vi "MALT132_0001.vi"() -> ()   [LabVIEW 2018]
uses:
  <instrlib>/AltonTech MALT/AltonTech MALT200817.lvlib
panel:
  in  "K1":bool
  in  "stop":bool
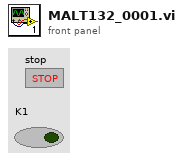
[diagram p1: front panel]
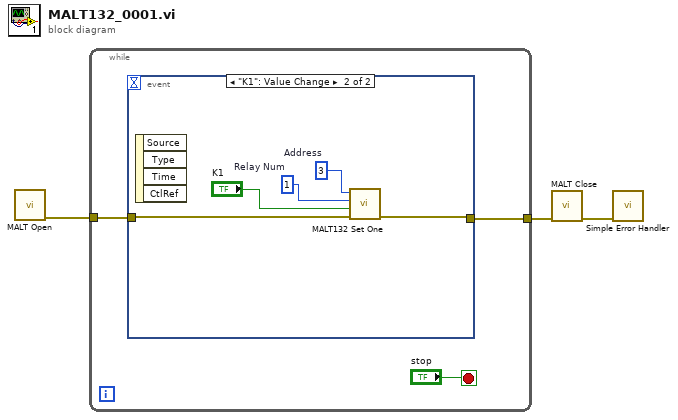
[diagram p0: block diagram]
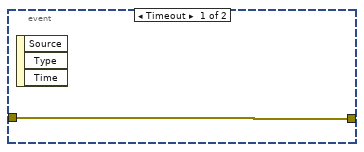
[diagram p2: hidden frame]
diagram:
  n1 = call <instrlib>:"MALT Open.vi"() -> ("error out"=w3:errorcluster)  [unwired: 11 in]
  n2 = while {
    tunnel: w3 -> [w5]
    tunnel: [w4] -> w2
    stop <- "stop" stop-if-true
    n3 = event shown="[1] \"K1\": Value Change" {
      selector: _ -> [_ _]
      dyn-events: _ -> [_ _]
      timeout: _ -> [_ _]
      tunnel: w5 -> [w7 w8]
      tunnel: [w7 w10] -> w4
      event Timeout {
        n4 = event-data() -> ()  [unwired: 1 in, 3 out]
      }
      event "K1": Value Change {
        w12 = 1  # Relay Num
        w11 = 3  # Address
        n5 = event-data() -> ()  [unwired: 1 in, 4 out]
        n6 = call <instrlib>:"MALT132 Set One.vi"("error in"=w8, "State"="K1", "Relay Num"=w12, "Address"=w11) -> ("error out"=w10:errorcluster)  [unwired: 7 in]
      }
    }
  }
  n7 = call <instrlib>:"MALT Close.vi"("error in"=w2) -> ("error out"=w1:errorcluster)  [unwired: 10 in]
  n8 = call <vilib>:"Simple Error Handler.vi"("error in (no error)"=w1) -> ()  [unwired: 4 in, 5 out]
